vi "best_score_ind.vi"(11 "Shape Report":T1(array[cluster])) -> (3 "Max Ind":i32)   [LabVIEW 2015]
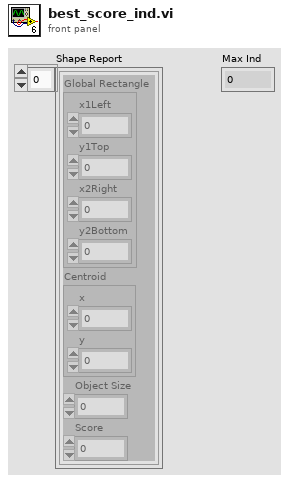
[diagram p1: front panel]
types:
  T1 = cluster{"Global Rectangle":cluster{"x1Left":i32, "y1Top":i32, "x2Right":i32, "y2Bottom":i32}, "Centroid":cluster{"x":sgl, "y":sgl}, "Object Size":u32, "Score":dbl}[]
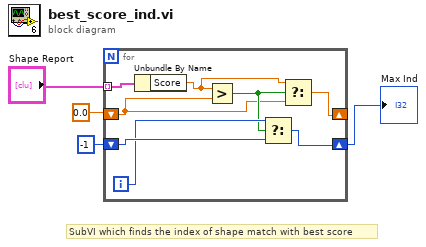
[diagram p0: block diagram]
diagram:
  # "SubVI which finds the index of shape match with best score"
  n1 = for {
    tunnel: "Shape Report" -> [w12] mode=indexing
    shift-right: [w5] -> _
    shift-left: 0.0 -> [w7]
    shift-right: [w9] -> w4
    shift-left: -1 -> [w11]
    i -> [w10]
    n2 = Unbundle By Name(w12) -> ("Score"=w6:dbl)
    n3 = Greater?(x=w6, y=w7) -> (0:w8:bool)
    n4 = Select(t=w10, s=w8, f=w11) -> (s? t:f=w9:i32)
    n5 = Select(t=w6, s=w8, f=w7) -> (s? t:f=w5:dbl)
  }
  "Max Ind" <- w4
